vi "toXML.vi"(8 "error in (no error)":errorcluster, 11 "Scan in":refnum<class "Scan.lvclass">) -> (0 "error out":errorcluster, 2 "xmlNode":refnum<class "xmlNode.lvclass">, 3 "Scan out":refnum<class "Scan.lvclass">)   [LabVIEW 2011, in "Tools.lvlib" / "Sequencing.lvlib" / "Scan.lvclass"]
uses:
  Scan.lvclass
  xmlNode/xmlNode.lvclass
  Point/Point.lvclass
  Scan.lvclass/Scan.ctl
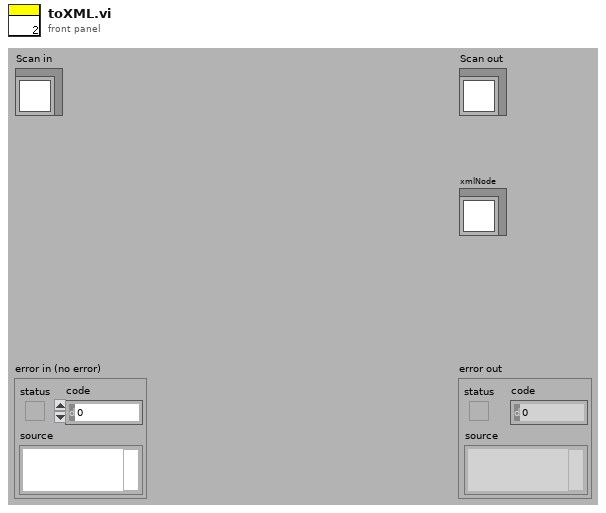
[diagram p1: front panel]
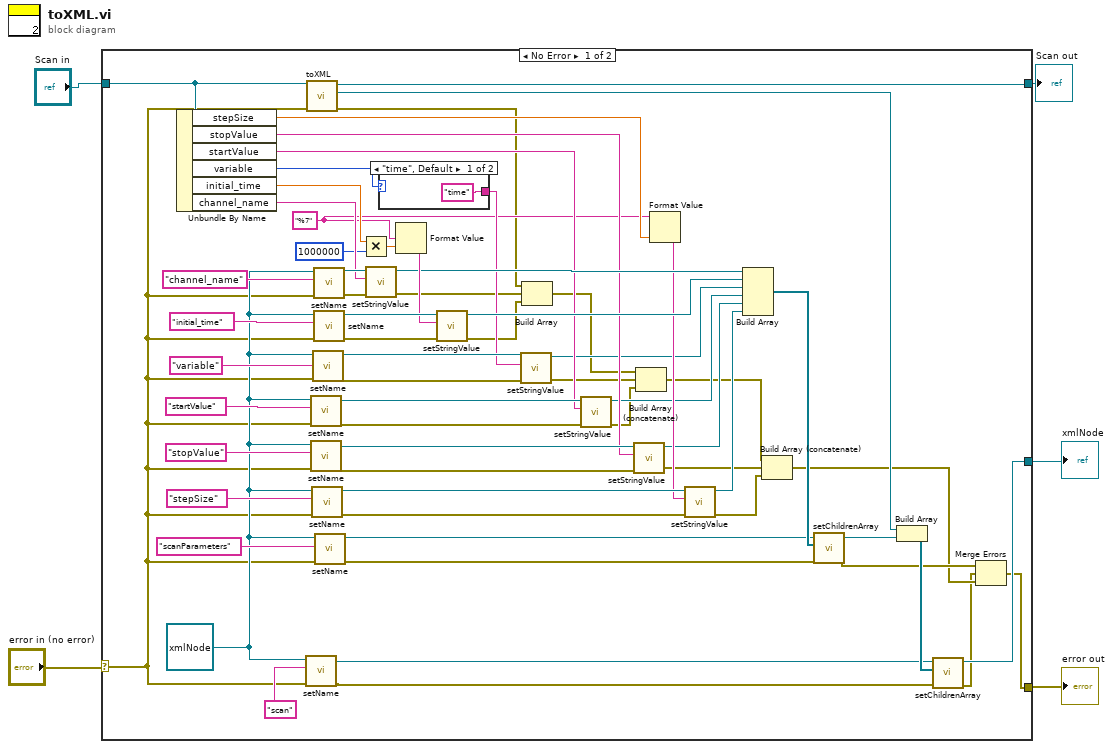
[diagram p0: block diagram]
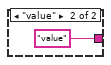
[diagram p2: hidden frame]
diagram:
  n1 = case shown="No Error" "error in (no error)" {
    selector: "error in (no error)" -> [w31 w72]
    tunnel: [w66 w73] -> w4
    tunnel: "Scan in" -> [w67 w73]
    tunnel: [w10 w72] -> w3
    tunnel: [w68 _] -> w1
    frame No Error {
      w35 = refnum<class "xmlNode.lvclass"> refnum ("Tools.lvlib:xml.lvlib:xmlNode.lvclass")
      w33 = "%7"
      n2 = Unbundle By Name(w67) -> ("stepSize"=w34:dbl, "stopValue"=w39:string, "startValue"=w43:string, "variable"=w50:enum16{"time", "value"}, "initial_time"=w59:dbl, "channel_name"=w62:string)
      n3 = call-dynamic "setName.vi"("error in (no error)"=w31, "name"="scan", "xmlNode.lvclass in"=w35) -> ("error out"=w21:errorcluster, "xmlNode.lvclass out"=w22:refnum<class "xmlNode.lvclass">)  [unwired: 7 in]
      n4 = call-parent "toXML.vi"("error in (no error)"=w31, "Point in"=w67) -> ("error out"=w8:errorcluster, "xmlNode"=w24:refnum<class "xmlNode.lvclass">, "Point out"=w66:refnum<class "Scan.lvclass">)  [unwired: 7 in]
      n5 = call-dynamic "setName.vi"("error in (no error)"=w31, "name"="startValue", "xmlNode.lvclass in"=w35) -> ("error out"=w44:errorcluster, "xmlNode.lvclass out"=w45:refnum<class "xmlNode.lvclass">)  [unwired: 7 in]
      n6 = call-dynamic "setName.vi"("error in (no error)"=w31, "name"="stopValue", "xmlNode.lvclass in"=w35) -> ("error out"=w40:errorcluster, "xmlNode.lvclass out"=w41:refnum<class "xmlNode.lvclass">)  [unwired: 7 in]
      n7 = call-dynamic "setName.vi"("error in (no error)"=w31, "name"="stepSize", "xmlNode.lvclass in"=w35) -> ("error out"=w36:errorcluster, "xmlNode.lvclass out"=w37:refnum<class "xmlNode.lvclass">)  [unwired: 7 in]
      n8 = call-dynamic "setName.vi"("error in (no error)"=w31, "name"="variable", "xmlNode.lvclass in"=w35) -> ("error out"=w48:errorcluster, "xmlNode.lvclass out"=w49:refnum<class "xmlNode.lvclass">)  [unwired: 7 in]
      n9 = call-dynamic "setName.vi"("error in (no error)"=w31, "name"="channel_name", "xmlNode.lvclass in"=w35) -> ("error out"=w63:errorcluster, "xmlNode.lvclass out"=w64:refnum<class "xmlNode.lvclass">)  [unwired: 7 in]
      n10 = call-dynamic "setName.vi"("error in (no error)"=w31, "name"="initial_time", "xmlNode.lvclass in"=w35) -> ("error out"=w60:errorcluster, "xmlNode.lvclass out"=w61:refnum<class "xmlNode.lvclass">)  [unwired: 7 in]
      n11 = call-dynamic "setName.vi"("error in (no error)"=w31, "name"="scanParameters", "xmlNode.lvclass in"=w35) -> ("error out"=w6:errorcluster, "xmlNode.lvclass out"=w7:refnum<class "xmlNode.lvclass">)  [unwired: 7 in]
      n12 = Multiply(x=w59, y=1000000) -> (x*y=w58:dbl)
      n13 = call-dynamic "setStringValue.vi"("error in (no error)"=w63, "stringValue"=w62, "xmlNode.lvclass in"=w64) -> ("error out"=w20:errorcluster, "xmlNode.lvclass out"=w53:refnum<class "xmlNode.lvclass">)  [unwired: 7 in]
      n14 = case shown="\"time\", Default" w50 {
        tunnel: ["time" "value"] -> w47
        frame "time", Default {
        }
        frame "value" {
        }
      }
      n15 = Format Value(format string=w33, value (0)=w58) -> (output string=w56:string)  [unwired: 1 in]
      n16 = call-dynamic "setStringValue.vi"("error in (no error)"=w60, "stringValue"=w56, "xmlNode.lvclass in"=w61) -> ("error out"=w19:errorcluster, "xmlNode.lvclass out"=w52:refnum<class "xmlNode.lvclass">)  [unwired: 7 in]
      n17 = call-dynamic "setStringValue.vi"("error in (no error)"=w48, "stringValue"=w47, "xmlNode.lvclass in"=w49) -> ("error out"=w17:errorcluster, "xmlNode.lvclass out"=w30:refnum<class "xmlNode.lvclass">)  [unwired: 7 in]
      n18 = Build Array(w8, w20, w19) -> (w18:errorcluster[])
      n19 = call-dynamic "setStringValue.vi"("error in (no error)"=w44, "stringValue"=w43, "xmlNode.lvclass in"=w45) -> ("error out"=w16:errorcluster, "xmlNode.lvclass out"=w29:refnum<class "xmlNode.lvclass">)  [unwired: 7 in]
      n20 = call-dynamic "setStringValue.vi"("error in (no error)"=w40, "stringValue"=w39, "xmlNode.lvclass in"=w41) -> ("error out"=w14:errorcluster, "xmlNode.lvclass out"=w28:refnum<class "xmlNode.lvclass">)  [unwired: 7 in]
      n21 = Build Array (concatenate)(w18, w17, w16) -> (w15:errorcluster[])
      n22 = Format Value(string ("")=w33, value (0)=w34) -> (output string=w32:string)  [unwired: 1 in]
      n23 = call-dynamic "setStringValue.vi"("error in (no error)"=w36, "stringValue"=w32, "xmlNode.lvclass in"=w37) -> ("error out"=w13:errorcluster, "xmlNode.lvclass out"=w27:refnum<class "xmlNode.lvclass">)  [unwired: 7 in]
      n24 = Build Array(w53, w52, w30, w29, w28, w27) -> (w26:refnum<class "xmlNode.lvclass">[])
      n25 = Build Array (concatenate)(w15, w14, w13) -> (w11:errorcluster[])
      n26 = call-dynamic "setChildrenArray.vi"("error in (no error)"=w6, "Children"=w26, "xmlNode.lvclass in"=w7) -> ("error out"=w12:errorcluster, "xmlNode.lvclass out"=w25:refnum<class "xmlNode.lvclass">)  [unwired: 7 in]
      n27 = Build Array(w24, w25) -> (w23:refnum<class "xmlNode.lvclass">[])
      n28 = call-dynamic "setChildrenArray.vi"("error in (no error)"=w21, "Children"=w23, "xmlNode.lvclass in"=w22) -> ("error out"=w9:errorcluster, "xmlNode.lvclass out"=w68:refnum<class "xmlNode.lvclass">)  [unwired: 7 in]
      n29 = Merge Errors(w12, w9, w11) -> (w10:errorcluster)
    }
    frame Error {
    }
  }
  "error out" <- w3
  "Scan out" <- w4
  "xmlNode" <- w1
